vi "Last Ack.vi"(10 "Alias":string, 11 "jettl Queue Actor in":refnum<class "jettl Queue Actor.lvclass">) -> (3 "jettl Queue Actor out":refnum<class "jettl Queue Actor.lvclass">)   [LabVIEW 2021, in "jettl.lvlib" / "jettl Queue Actor.lvclass"]
uses:
  jettl Queue Actor.lvclass
  jettl Queue Actor.lvclass/jettl Queue Actor.ctl
  jettl.lvlib
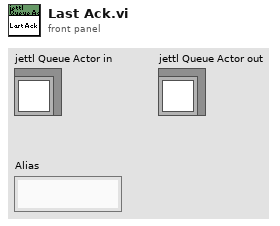
[diagram p1: front panel]
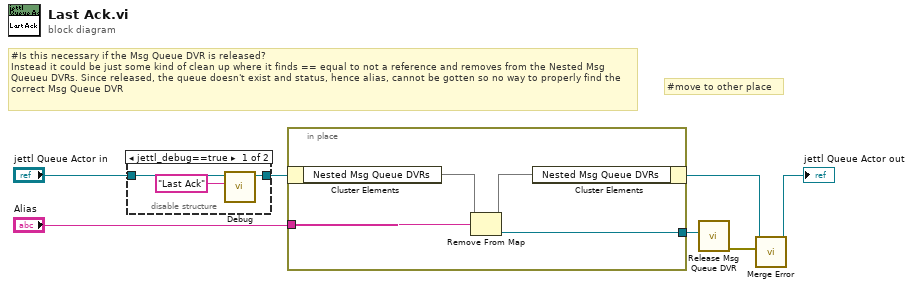
[diagram p0: block diagram]
diagram:
  # "#Is this necessary if the Msg Queue DVR is released?\nInstead it could be just some kind of clean up where it finds == equal to not a reference and removes from the Nested Msg Queueu DVRs. Since released, the queue doesn't exist and status, hence alias, cannot be gotten so no way to properly find the correct Msg Queue DVR"
  # "#move to other place"
  n1 = disable-structure shown="jettl_debug==true" {
    disable-tunnel: "jettl Queue Actor in" -> [w10 w11]
    disable-tunnel: [w9 w11] -> w2
    frame condition #0 (active) {
      n2 = call "Debug.vi"("Method"="Last Ack", "jettl Queue Actor in"=w10) -> ("jettl Queue Actor out"=w9:refnum<class "jettl Queue Actor.lvclass">)  [unwired: 9 in]
    }
    frame condition #1 {
    }
  }
  n3 = in-place {
    in-place-border: "Alias" -> [w14]
    in-place-border: [w13] -> w7
    n4 = in-place-cluster #1(w2) -> ("Nested Msg Queue DVRs"=w15:map{string, refnum<data-value>})
    n5 = Remove From Map(10:w14, 11:w15) -> (1:w13:refnum<data-value>, 3:w12:map{string, refnum<data-value>})  [unwired: 1 out]
    n6 = in-place-cluster #1("Nested Msg Queue DVRs"=w12) -> (w5:refnum<class "jettl Queue Actor.lvclass">)
  }
  n7 = call "Release Msg Queue DVR.vi"("Msg Queue DVR"=w7) -> ("error out"=w6:errorcluster)  [unwired: 10 in]
  n8 = call-dynamic "Merge Error.vi"("Error"=w6, "jettl Queue Actor in"=w5) -> ("jettl Queue Actor out"=→"jettl Queue Actor out":refnum<class "jettl Queue Actor.lvclass">)  [unwired: 9 in]
